vi "计时（记录按钮点击的时间间隔）.vi"() -> ()   [LabVIEW 2014]
panel:
  in  "确定":bool
  out "Elapsed Time (s)":dbl caption="已用时间(s)"
  in  "停止":bool
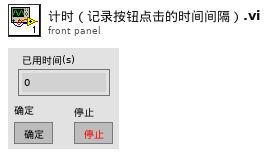
[diagram p1: front panel]
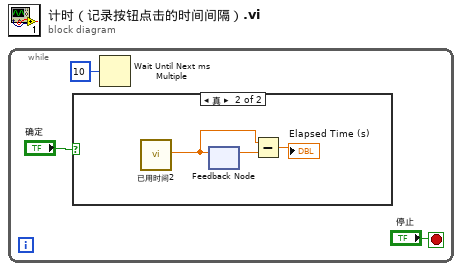
[diagram p0: block diagram]
diagram:
  n1 = while {
    stop <- "停止" stop-if-true
    n2 = case shown="真" "确定" {
      frame False {
      }
      frame True {
        n3 = call "已用时间2"() -> ("Elapsed Time (s)"=w4:dbl)  [unwired: 12 in, 7 out]
        n4 = feedback #1() -> (w5:dbl)  [unwired: 1 in]
        n5 = feedback-in #1(w4) -> ()
        n6 = Subtract(x=w4, y=w5) -> (x-y=→"Elapsed Time (s)":dbl)
      }
    }
    n7 = Wait Until Next ms Multiple(millisecond multiple=u32 10 ("毫秒倍数")) -> ()  [unwired: 1 out]
  }
